vi "Start Logging.vi"(8 "error in (no error)":errorcluster, 10 "Path":path, 11 "Data Logger Interface in":refnum<class "TDMS Data Logger Actor.lvclass">) -> (0 "error out":errorcluster, 3 "Data Logger Interface out":refnum<class "TDMS Data Logger Actor.lvclass">)   [LabVIEW 2024, in "TDMS Data Logger Actor.lvlib" / "TDMS Data Logger Actor.lvclass"]
uses:
  TDMS Data Logger Actor.lvclass
  C:/Program Files (x86)/National Instruments/LabVIEW 2024/vi.lib/ActorFramework/Actor/Actor.lvclass
  TDMS Data Logger Actor.lvclass/TDMS Data Logger Actor.ctl
  <vilib>/ActorFramework/Actor/Actor.lvclass/Actor.ctl
  <vilib>/ActorFramework/Message Enqueuer/Message Enqueuer.lvclass/Message Enqueuer.ctl
  <vilib>/ActorFramework/Message Enqueuer/Enqueue.vi
  Data Logger Actor Reply Interface/Data Logger Actor Reply Interface Messages/Logging Active Msg/Logging Active Msg.lvclass
  C:/Program Files (x86)/National Instruments/LabVIEW 2024/vi.lib/ActorFramework/Message/Message.lvclass
  <vilib>/ActorFramework/Message Priority Queue/Priority Enqueue.vi
  <vilib>/ActorFramework/Actor/Actor.lvclass
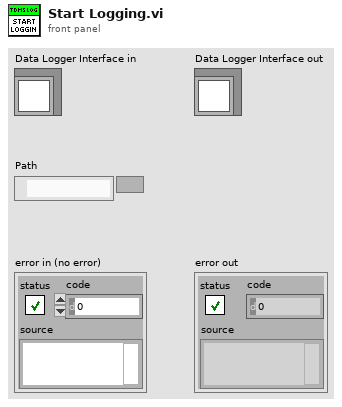
[diagram p1: front panel]
types:
  T1 = enum16{"open", "open or create", "create or replace", "create", "open (read-only)"}
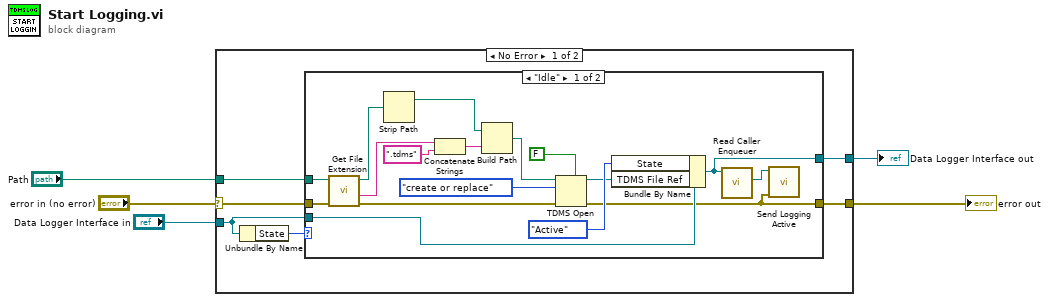
[diagram p0: block diagram]
diagram:
  n1 = case shown="No Error" "error in (no error)" {
    selector: "error in (no error)" -> [w8 w31]
    tunnel: "Data Logger Interface in" -> [w10 w32]
    tunnel: [w9 w32] -> w3
    tunnel: [w7 w31] -> w2
    tunnel: "Path" -> [w6 _]
    frame No Error {
      n2 = Unbundle By Name(w10) -> ("State"=w11:enum16{"Idle", "Active", "Paused"})
      n3 = case shown="\"Idle\"" w11 {
        tunnel: w10 -> [w27 w30]
        tunnel: [w25 w30] -> w9
        tunnel: w8 -> [w15 w29]
        tunnel: [w13 w29] -> w7
        tunnel: w6 -> [w22 _]
        frame "Idle" {
          n4 = call <vilib>:"Get File Extension.vi"("error in (no error)"=w15, "file"=w22) -> ("error out"=w14:errorcluster, "filename without extension"=w19:string, "dup file"=w21:path)  [unwired: 5 in, 2 out]
          n5 = Strip Path(path=w21) -> (stripped path=w20:path)  [unwired: 1 out]
          n6 = Concatenate Strings(w19, ".tdms" ("string")) -> (w17:string)
          n7 = Build Path(base path=w20, name or relative path=w17) -> (appended path=w16:path)
          n8 = TDMS Open(5:FALSE ("create index file? (T)"), 8:w14, 10:T1."create or replace" ("operation (0:open)"), 11:w16) -> (0:w13:errorcluster, 3:w23:refnum<k34>)  [unwired: 3 in]
          n9 = Bundle By Name(cluster=w27, "State"=enum16{"Idle", "Active", "Paused"}."Active", "TDMS File Ref"=w23) -> (w25:refnum<class "TDMS Data Logger Actor.lvclass">)
          n10 = call <vilib>:"Read Caller Enqueuer.vi"("Actor"=w25) -> ("Caller Enqueuer"=w28:refnum<class "Message Enqueuer.lvclass">)  [unwired: 10 in]
          n11 = call "Send Logging Active.vi"("error in (no error)"=w13, "Message Enqueuer"=w28) -> ()  [unwired: 8 in, 2 out]
        }
        frame Default {
        }
      }
    }
    frame Error {
    }
  }
  "error out" <- w2
  "Data Logger Interface out" <- w3
